vi "ConfigSMU2ch_voltage.vi"(0 "IVI Refnum in":refnum<k15>, 1 "Channel DxSupply":string="0", 2 "Voltage Level DxSupply":dbl, 3 "Current Limit DxSupply":dbl, 11 "error in (no error)":errorcluster, 12 "Channel DxBoot0":string="0", 13 "Voltage Level DxBoot0":dbl, 14 "Current Limit DxBoot0":dbl) -> (4 "IVI Refnum out":refnum<k15>, 15 "error out":errorcluster)   [LabVIEW 2018]
uses:
  <instrlib>/niDCPower/nidcpower.llb/niDCPower Output Function.ctl
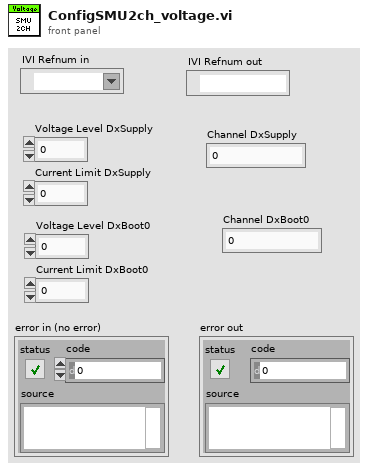
[diagram p1: front panel]
types:
  T1 = typedef "niDCPower Output Function.ctl" = i32
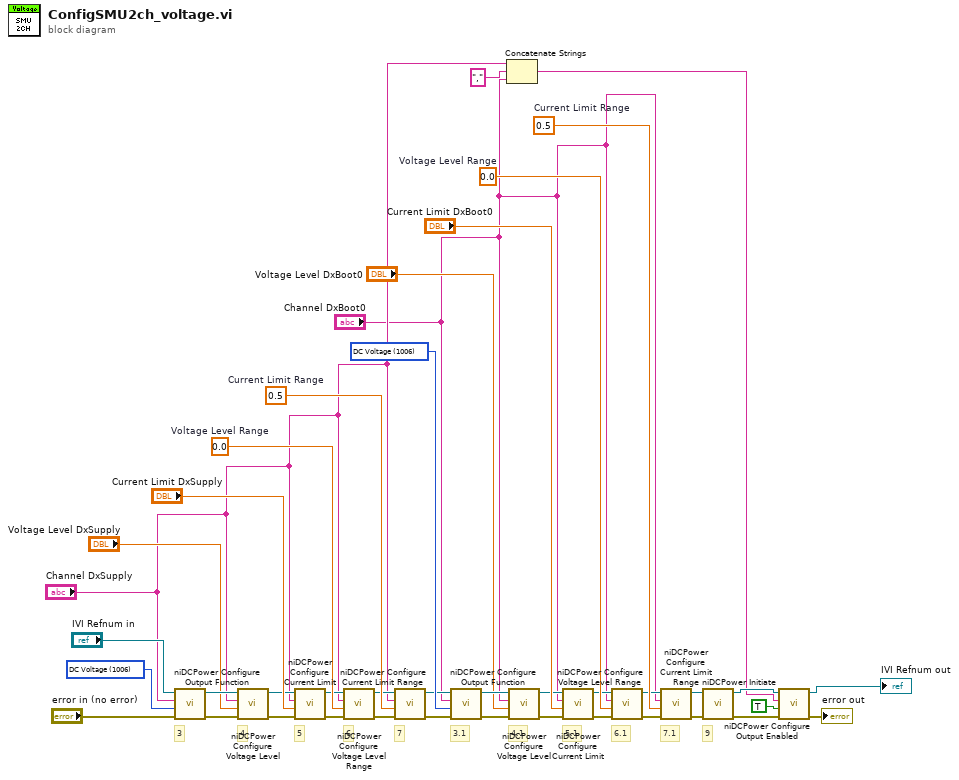
[diagram p0: block diagram]
diagram:
  w20 = 0.0  # Voltage Level Range
  w21 = 0.5  # Current Limit Range
  w24 = T1 1006 items=["DC Voltage"=1006, "DC Current"=1007, "Pulse Voltage"=1049, "Pulse Current"=1050] ("output function")
  w37 = 0.0  # Voltage Level Range
  w38 = 0.5  # Current Limit Range
  w41 = T1 1006 items=["DC Voltage"=1006, "DC Current"=1007, "Pulse Voltage"=1049, "Pulse Current"=1050] ("output function")
  # "7.1"
  # "6.1"
  # "3.1"
  # "5.1"
  # "4.1"
  # "9"
  # "7"
  # "6"
  # "3"
  # "5"
  # "4"
  n1 = call <instrlib>:"niDCPower Configure Output Function.vi"("error in (no error)"="error in (no error)", "output function"=w41, "channel name"="Channel DxSupply", "instrument handle"="IVI Refnum in") -> ("error out"=w40:errorcluster, "instrument handle out"=w39:refnum<k15>)  [unwired: 6 out]
  n2 = call <instrlib>:"niDCPower Configure Voltage Level.vi"("error in (no error)"=w40, "voltage level"="Voltage Level DxSupply", "channel name"="Channel DxSupply", "instrument handle"=w39) -> ("error out"=w30:errorcluster, "instrument handle out"=w29:refnum<k15>)  [unwired: 6 out]
  n3 = call <instrlib>:"niDCPower Configure Current Limit.vi"("error in (no error)"=w30, "current limit"="Current Limit DxSupply", "channel name"="Channel DxSupply", "instrument handle"=w29) -> ("error out"=w33:errorcluster, "instrument handle out"=w34:refnum<k15>)  [unwired: 1 in, 5 out]
  n4 = call <instrlib>:"niDCPower Configure Voltage Level Range.vi"("error in (no error)"=w33, "voltage level range"=w37, "channel name"="Channel DxSupply", "instrument handle"=w34) -> ("error out"=w35:errorcluster, "instrument handle out"=w36:refnum<k15>)  [unwired: 6 out]
  n5 = call <instrlib>:"niDCPower Configure Current Limit Range.vi"("error in (no error)"=w35, "current limit range"=w38, "channel name"="Channel DxSupply", "instrument handle"=w36) -> ("error out"=w10:errorcluster, "instrument handle out"=w11:refnum<k15>)  [unwired: 6 out]
  n6 = call <instrlib>:"niDCPower Configure Output Function.vi"("error in (no error)"=w10, "output function"=w24, "channel name"="Channel DxBoot0", "instrument handle"=w11) -> ("error out"=w23:errorcluster, "instrument handle out"=w22:refnum<k15>)  [unwired: 6 out]
  n7 = Concatenate Strings("Channel DxSupply", "," ("string"), "Channel DxBoot0") -> (w3:string)
  n8 = call <instrlib>:"niDCPower Configure Voltage Level.vi"("error in (no error)"=w23, "voltage level"="Voltage Level DxBoot0", "channel name"="Channel DxBoot0", "instrument handle"=w22) -> ("error out"=w13:errorcluster, "instrument handle out"=w12:refnum<k15>)  [unwired: 6 out]
  n9 = call <instrlib>:"niDCPower Configure Current Limit.vi"("error in (no error)"=w13, "current limit"="Current Limit DxBoot0", "channel name"="Channel DxBoot0", "instrument handle"=w12) -> ("error out"=w16:errorcluster, "instrument handle out"=w17:refnum<k15>)  [unwired: 1 in, 5 out]
  n10 = call <instrlib>:"niDCPower Configure Voltage Level Range.vi"("error in (no error)"=w16, "voltage level range"=w20, "channel name"="Channel DxBoot0", "instrument handle"=w17) -> ("error out"=w18:errorcluster, "instrument handle out"=w19:refnum<k15>)  [unwired: 6 out]
  n11 = call <instrlib>:"niDCPower Configure Current Limit Range.vi"("error in (no error)"=w18, "current limit range"=w21, "channel name"="Channel DxBoot0", "instrument handle"=w19) -> ("error out"=w1:errorcluster, "instrument handle out"=w2:refnum<k15>)  [unwired: 6 out]
  n12 = call <instrlib>:"niDCPower Initiate.vi"("error in (no error)"=w1, "instrument handle"=w2) -> ("error out"=w6:errorcluster, "instrument handle out"=w7:refnum<k15>)  [unwired: 2 in, 6 out]
  n13 = call <instrlib>:"niDCPower Configure Output Enabled.vi"("error in (no error)"=w6, "output enabled"=TRUE, "channel name"=w3, "instrument handle"=w7) -> ("error out"=→"error out":errorcluster, "instrument handle out"=→"IVI Refnum out":refnum<k15>)  [unwired: 6 in]
